vi "Get Nth Line.vi"(8 "error in (no error)":errorcluster, 10 "line index":u32, 11 "String in":refnum<class "String.lvclass">) -> (0 "error out":errorcluster, 1 "position of line start":u32, 2 "line text":string, 3 "String out":refnum<class "String.lvclass">, 4 "position of line end":u32)   [LabVIEW 2020, in "String.lvclass"]
doc: "Gets the characters that make up the Nth line in a string control and returns the offsets in the original string in bytes.\n\n You can use this method to determine how the text in a string control is word-wrapped. The position indexes are byte indexes. These are usually equivalent to character indexes, except when using text that has characters that use multiple bytes, such as Asian character sets.\n\n Example\n\nQControl Class wrapper around the <b>String : Get Nth Line Method</b>.\n<b> </b> <b> </b>\n©2016 Q Software Innovations, LLC (QSI)\nwritten by Quentin Alldredge\nproduced in LabVIEW 2015\n\nsupport@qsoftwareinnovations.com\nwww.qsoftwareinnovations.com\n\nAll rights reserved.\n\nRedistribution and use in source and binary forms, with or without modification, are permitted provided that the following conditions are met:\n\n * Redistributions of source code must retain the above copyright notice, this list of conditions and the following disclaimer.\n * Redistributions in binary form must reproduce the above copyright notice, this list of conditions and the following disclaimer in the documentation and/or other materials provided with the distribution.\n * Neither the name of Q Software Innovations, LLC. nor the names of its contributors may be used to endorse or promote products derived from this software without specific prior written permission.\n\nTHIS SOFTWARE IS PROVIDED BY THE COPYRIGHT HOLDERS AND CONTRIBUTORS \"AS IS\" AND ANY EXPRESS OR IMPLIED WARRANTIES, INCLUDING, BUT NOT LIMITED TO, THE IMPLIED WARRANTIES OF MERCHANTABILITY AND FITNESS FOR A PARTICULAR PURPOSE ARE DISCLAIMED. IN NO EVENT SHALL THE COPYRIGHT OWNER OR CONTRIBUTORS BE LIABLE FOR ANY DIRECT, INDIRECT, INCIDENTAL, SPECIAL, EXEMPLARY, OR CONSEQUENTIAL DAMAGES (INCLUDING, BUT NOT LIMITED TO, PROCUREMENT OF SUBSTITUTE GOODS OR SERVICES; LOSS OF USE, DATA, OR PROFITS; OR BUSINESS INTERRUPTION) HOWEVER CAUSED AND ON ANY THEORY OF LIABILITY, WHETHER IN CONTRACT, STRICT LIABILITY, OR TORT (INCLUDING NEGLIGENCE OR OTHERWISE) ARISING IN ANY WAY OUT OF THE USE OF THIS SOFTWARE, EVEN IF ADVISED OF THE POSSIBILITY OF SUCH DAMAGE."
uses:
  String.lvclass
  String.lvclass/String.ctl
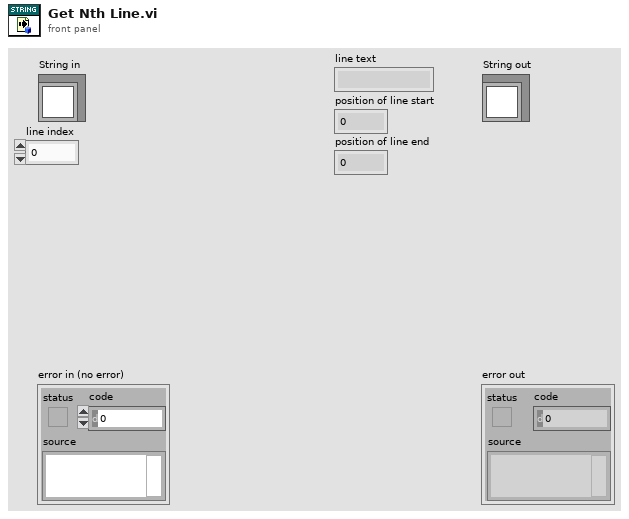
[diagram p1: front panel]
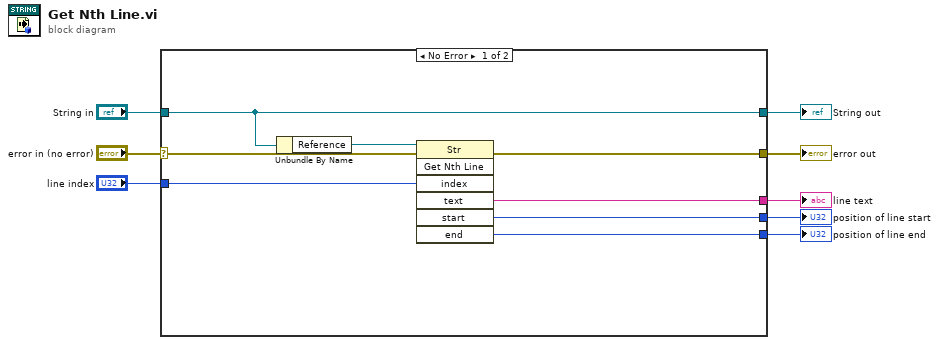
[diagram p0: block diagram]
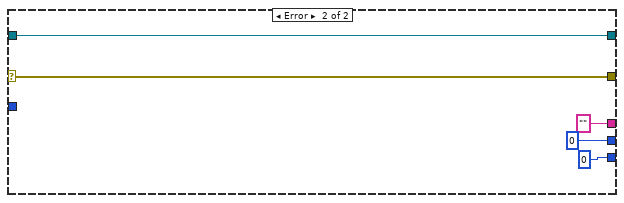
[diagram p2: hidden frame]
diagram:
  n1 = case shown="No Error" "error in (no error)" {
    selector: "error in (no error)" -> [w16 w21]
    tunnel: [w15 w21] -> w7
    tunnel: [w14 w20] -> w5
    tunnel: "String in" -> [w14 w20]
    tunnel: "line index" -> [w12 _]
    tunnel: [w11 "" ("text")] -> w3
    tunnel: [w10 u32 0 ("start")] -> w2
    tunnel: [w9 u32 0 ("end")] -> w1
    frame No Error {
      n2 = Unbundle By Name(w14) -> ("Reference"=w13:refnum<vi>)
      n3 = invoke class="Str" method="Get Nth Line"(reference=w13, error in=w16, "index"=w12) -> (error out=w15:errorcluster, "text"=w11:string, "start"=w10:u32, "end"=w9:u32)  [unwired: 4 in, 3 out]
    }
    frame Error {
    }
  }
  "error out" <- w7
  "String out" <- w5
  "line text" <- w3
  "position of line start" <- w2
  "position of line end" <- w1
